vi "relogon.vi"(3 "relogon":bool, 4 "data server address in":string, 5 "Connection ID":refnum<k5>) -> (2 "connection ID out":refnum<k5>)   [LabVIEW 2012]
panel:
  out "error out":errorcluster
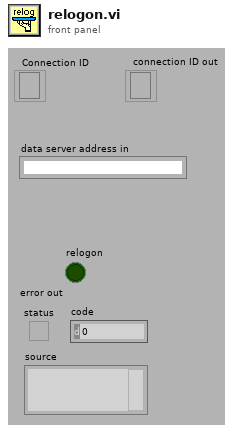
[diagram p1: front panel]
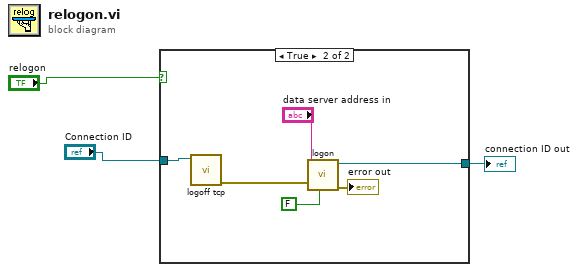
[diagram p0: block diagram]
diagram:
  n1 = case shown="True" "relogon" {
    tunnel: "Connection ID" -> [w4 w8]
    tunnel: [w4 w7] -> w1
    frame False {
    }
    frame True {
      n2 = call "logoff tcp.vi"("Connection ID"=w8) -> ("error out"=w9:errorcluster)  [unwired: 9 in, 1 out]
      n3 = call "logon.vi"("Display error messages?"=FALSE, "error in"=w9, "data server address in"="data server address in") -> ("error out"=→"error out":errorcluster, "connection ID"=w7:refnum<k5>)  [unwired: 5 in, 2 out]
    }
  }
  "connection ID out" <- w1
